vi "Strafe Null Rotation.vi"(6 "Deadzone":dbl=0.15 format="%#_13g", 7 "Gyro gains":T1={"proportional gain (Kc)"=-0.01, "integral time (Ti, min)"=0.0, "derivative time (Td, min)"=0.0} {"derivative time (Td, min)" format="%.3f"; "integral time (Ti, min)" format="%.3f"; "proportional gain (Kc)" min=-10.0 max=10.0 step=0.0001 format="%.3f"}, 8 "error in (no error)":errorcluster, 9 "Gyro Angle":dbl, 10 "Strafe (Left Joystick X)":dbl, 11 "Rotation (Right Joystick X)":dbl) -> (0 "error out":errorcluster, 1 "In deadzone?":bool=TRUE, 3 "Rotation":dbl=0.007874015748031496)   [LabVIEW 2014]
doc: "Nullify any torque from strafing by counter-rotating the drive wheels.\nMeasures rotation with gyro angle."
uses:
  <vilib>/addons/control/pid/pid.llb/PID (DBL).vi
  <vilib>/addons/control/pid/NI_PID_pid.lvlib
panel:
  in  "output range":cluster{"output high":dbl, "output low":dbl}={"output high"=0.5, "output low"=-0.5}
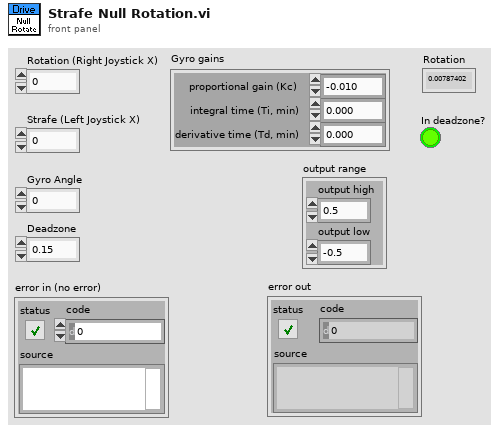
[diagram p1: front panel]
types:
  T1 = cluster{"proportional gain (Kc)":dbl, "integral time (Ti, min)":dbl, "derivative time (Td, min)":dbl}
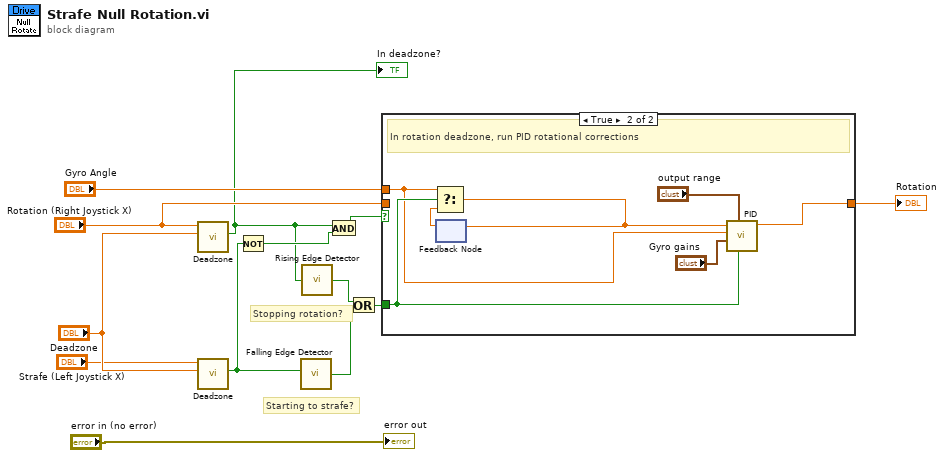
[diagram p0: block diagram]
diagram:
  # "Stopping rotation?"
  # "Starting to strafe?"
  n1 = call "Deadzone.vi"("Deadzone"="Deadzone", "Input"="Rotation (Right Joystick X)") -> ("In deadzone?"=w4:bool)  [unwired: 7 in, 2 out]
  "In deadzone?" <- w4
  n2 = call "Deadzone.vi"("Deadzone"="Deadzone", "Input"="Strafe (Left Joystick X)") -> ("In deadzone?"=w6:bool)  [unwired: 7 in, 2 out]
  n3 = Not(x=w6) -> (.not. x?=w5:bool)
  n4 = call "Falling Edge Detector.vi"("Input"=w6) -> ("Falling edge?"=w2:bool)
  n5 = call "Rising Edge Detector.vi"("Input"=w4) -> ("Rising edge?"=w3:bool)
  n6 = And(x=w4, y=w5) -> (x .and. y?=w7:bool)
  n7 = Or(x=w3, y=w2) -> (x .or. y?=w1:bool)
  n8 = case shown="True" w7 {
    tunnel: w1 -> [_ w19]
    tunnel: [w14 w16] -> w12
    tunnel: "Gyro Angle" -> [_ w15]
    tunnel: "Rotation (Right Joystick X)" -> [w14 _]
    frame False {
      # "Out of rotation deadzone, no rotational corrections"
    }
    frame True {
      # "In rotation deadzone, run PID rotational corrections"
      n9 = feedback #1() -> (w18:dbl)  [unwired: 1 in]
      n10 = Select(t=w15, s=w19, f=w18) -> (s? t:f=w17:dbl)
      n11 = feedback-in #1(w17) -> ()
      n12 = call-poly <vilib>:"PID.vi"("reinitialize? (F)"=w19, "output range"="output range", "PID gains"="Gyro gains", "process variable"=w15, "setpoint"=w17) -> ("output"=w16:dbl)  [unwired: 5 in, 1 out]
    }
  }
  "Rotation" <- w12
  "error out" <- "error in (no error)"
